vi "LVClass_CorrectionDataManager GetActuatorInluence.vi"(0 "CorrectionDataManager in":refnum<class "CorrectionDataManager.lvclass">, 5 "N° actuator":i32, 7 "Use actuator pupil ?":bool, 9 "Influence HasoSlopes":refnum<class "HasoSlopes.lvclass">, 11 "error in (no error)":errorcluster) -> (4 "CorrectionDataManager out":refnum<class "CorrectionDataManager.lvclass">, 10 "Influence HasoSlopes (dup)":refnum<class "HasoSlopes.lvclass">, 15 "error out":errorcluster)   [LabVIEW 2020, in "CorrectionDataManager.lvclass"]
doc: "Get experiment command applied for calibration steps count index.\n\n--------------------------------------------------------------------------------\n\n<B>corrdata_managerIn </B> : CorrDataManager object.\n<B>corrdata_managerOut </B> : CorrDataManager object.\n<B>index </B> : Index of the calibration step.\n<B>commands </B> : Wavefront corrector commands associated to the index calibration step.\n<B>ErrorIn </B> : Error\n<B>ErrorOut </B> : Error\n\n--------------------------------------------------------------------------------"
uses:
  CorrectionDataManager.lvclass
  HasoSlopes.lvclass
  CorrectionDataManager.lvclass/CorrectionDataManager.ctl
  LVClass_HasoSlopes Read HasoSlopes _ property.vi
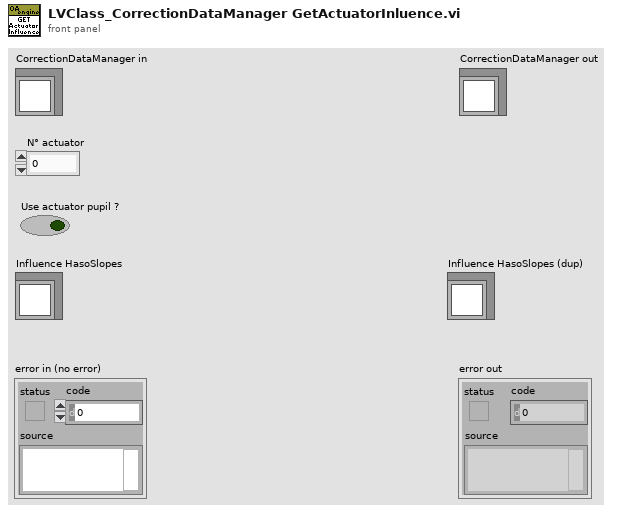
[diagram p1: front panel]
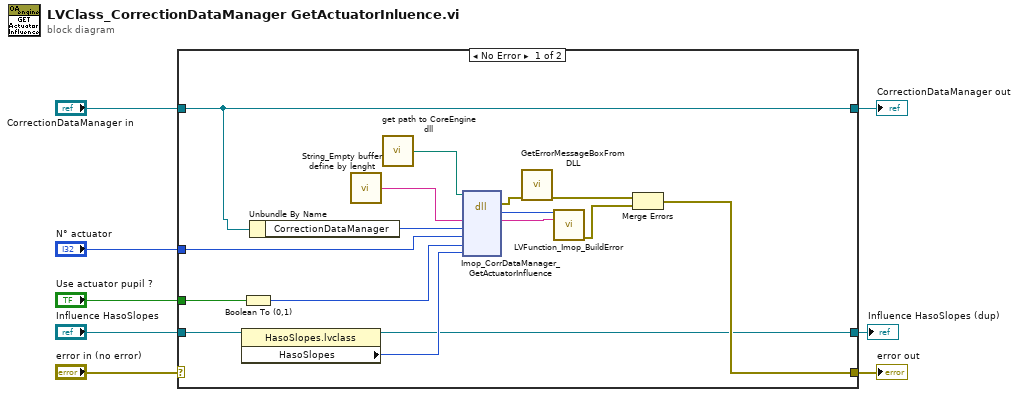
[diagram p0: block diagram]
diagram:
  n1 = case shown="No Error" "error in (no error)" {
    selector: "error in (no error)" -> [_ w27]
    tunnel: [w17 w27] -> w8
    tunnel: [w15 w26] -> w7
    tunnel: "CorrectionDataManager in" -> [w15 w26]
    tunnel: "N° actuator" -> [w14 _]
    tunnel: "Use actuator pupil ?" -> [w11 _]
    tunnel: "Influence HasoSlopes" -> [w13 w25]
    tunnel: [w9 w25] -> w1
    frame No Error {
      n2 = property class="HasoSlopes.lvclass"(reference=w13) -> (reference out=w9:refnum<class "HasoSlopes.lvclass">, "HasoSlopes"=w12:i32)  [unwired: 1 in, 1 out]
      n3 = Boolean To (0,1)(Boolean=w11) -> (0, 1=w10:i16)
      n4 = Unbundle By Name(w15) -> ("CorrectionDataManager"=w16:i32)
      n5 = call "String_Empty buffer define by lenght.vi"() -> ("Empty buffer"=w22:string)  [unwired: 1 in]
      n6 = call "get path to CoreEngine dll.vi"() -> ("path to c_interface_vc100.dll"=w21:path)  [unwired: 12 in, 3 out]
      n7 = dll-call lib="D:/FLE/0.Code/CoreEngine4_Suite/LV2011_interface/DLLs/c_interface_vc100.dll" fn="Imop_CorrDataManager_GetActuatorInfluence"(path in=w21, "message"=w22, "corrdata_manager"=w16, "experience_index"=w14, "Use actuator Pupil"=w10, "Influence HasoSlopes"=w12) -> (error out=w20:errorcluster, "return type"=w24:i32, "message"=w23:string)  [unwired: 6 in, 1 out]
      n8 = call "GetErrorMessageBoxFromDLL.vi"("error IN"=w20) -> ("error OUT"=w19:errorcluster)  [unwired: 10 in]
      n9 = call "LVFunction_Imop_BuildError.vi"("code"=w24, "String to Prepend to source (\"\")"=w23) -> ("error out"=w18:errorcluster)  [unwired: 13 in]
      n10 = Merge Errors(w19, w18) -> (w17:errorcluster)
    }
    frame Error {
    }
  }
  "error out" <- w8
  "CorrectionDataManager out" <- w7
  "Influence HasoSlopes (dup)" <- w1
